vi "LC_Relay_Protection_R2.vi"(0 "Protection settings":T4, 1 "Reset Relay":bool, 3 "RMS minimum\nvalues":cluster{"VRMS values":dbl, "IRMS values":dbl}, 5 "RMS values":dbl[](array[numeric]), 9 "Total power values":dbl[](array[numeric]), 11 "input cluster":T3, 12 "Blocking in":bool, 14 "Transfer Trip":bool) -> (4 "trip signal":bool, 6 "Reclose":bool, 8 "Relay state":cluster{"Lockout":bool, "State":i16}, 10 "Blocking out":bool[](array[boolean]), 15 "output cluster":T3)   [LabVIEW 2016]
doc: "Modified LC_Relay_Protection for Relay2"
uses:
  <vilib>/addons/Electrical Power/Protection/Definite Time Delay/subVIs/fpga_Timer Feedback Var.ctl
  <vilib>/addons/Electrical Power/Protection/Definite Time Delay/subVIs/fpga_State.ctl
  <vilib>/addons/Electrical Power/Protection/Inverse Time Delay/subVIs/ep_Operate Time.ctl
  <vilib>/addons/Electrical Power/Protection/NI_EP_Protection.lvlib
  <vilib>/addons/Electrical Power/Protection/NI_EP_Protection_FPGA.lvlib
panel:
  out "VR error":i32
  out "I error":i32
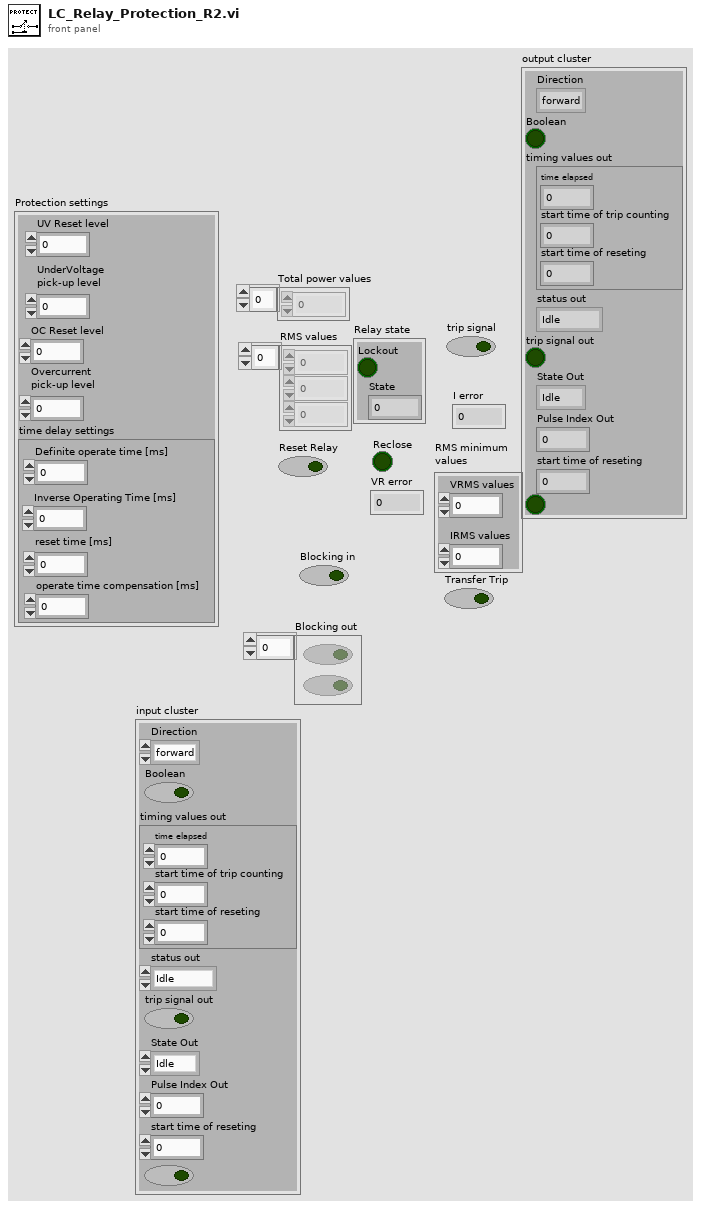
[diagram p1: front panel]
types:
  T1 = typedef "NI_EP_Protection_FPGA.lvlib/fpga_Timer Feedback Var.ctl" = cluster{"time elapsed":u32, "start time of trip counting":u32, "start time of reseting":u32}
  T2 = typedef "NI_EP_Protection_FPGA.lvlib/fpga_State.ctl" = enum16{"Idle", "Trip Counting", "Tripped", "Reset Counting"}
  T3 = cluster{"Direction":enum16{"forward", "backward", "N/D"}, "Boolean":bool, "timing values out":T1, "status out":T2, "trip signal out":bool, "State Out":enum16{"Idle", "Wait for Trip", "PulseClosing", "Locked"}, "Pulse Index Out":i32, "start time of reseting":u32, bool}
  T4 = cluster{"UV Reset level":dbl, "UnderVoltage \npick-up level":dbl, "OC Reset level":dbl, "Overcurrent\npick-up level":dbl, "time delay settings":cluster{"Definite operate time [ms]":u32, "Inverse Operating Time [ms]":u32, "reset time [ms]":u32, "operate time compensation [ms]":u32}}
  T5 = enum16{"Idle", "Wait for Trip", "PulseClosing", "Locked"}
  T6 = cluster{"Definite operate time [ms]":u32, "Inverse Operating Time [ms]":u32, "reset time [ms]":u32, "operate time compensation [ms]":u32}
  T7 = typedef "NI_EP_Protection.lvlib/ep_Operate Time.ctl" = cluster{"A [s]":dbl, "B [s]":dbl, "alpha":dbl, "K2 [s]":dbl, "K1 [s]":dbl, "K3 [s]":dbl}
  T8 = cluster{u32, "reset time [ms]":u32, "reset time [ms]":u32}
  T9 = cluster{"Definite operate time [ms]":u32, "reset time [ms]":u32, "reset time [ms]":u32}
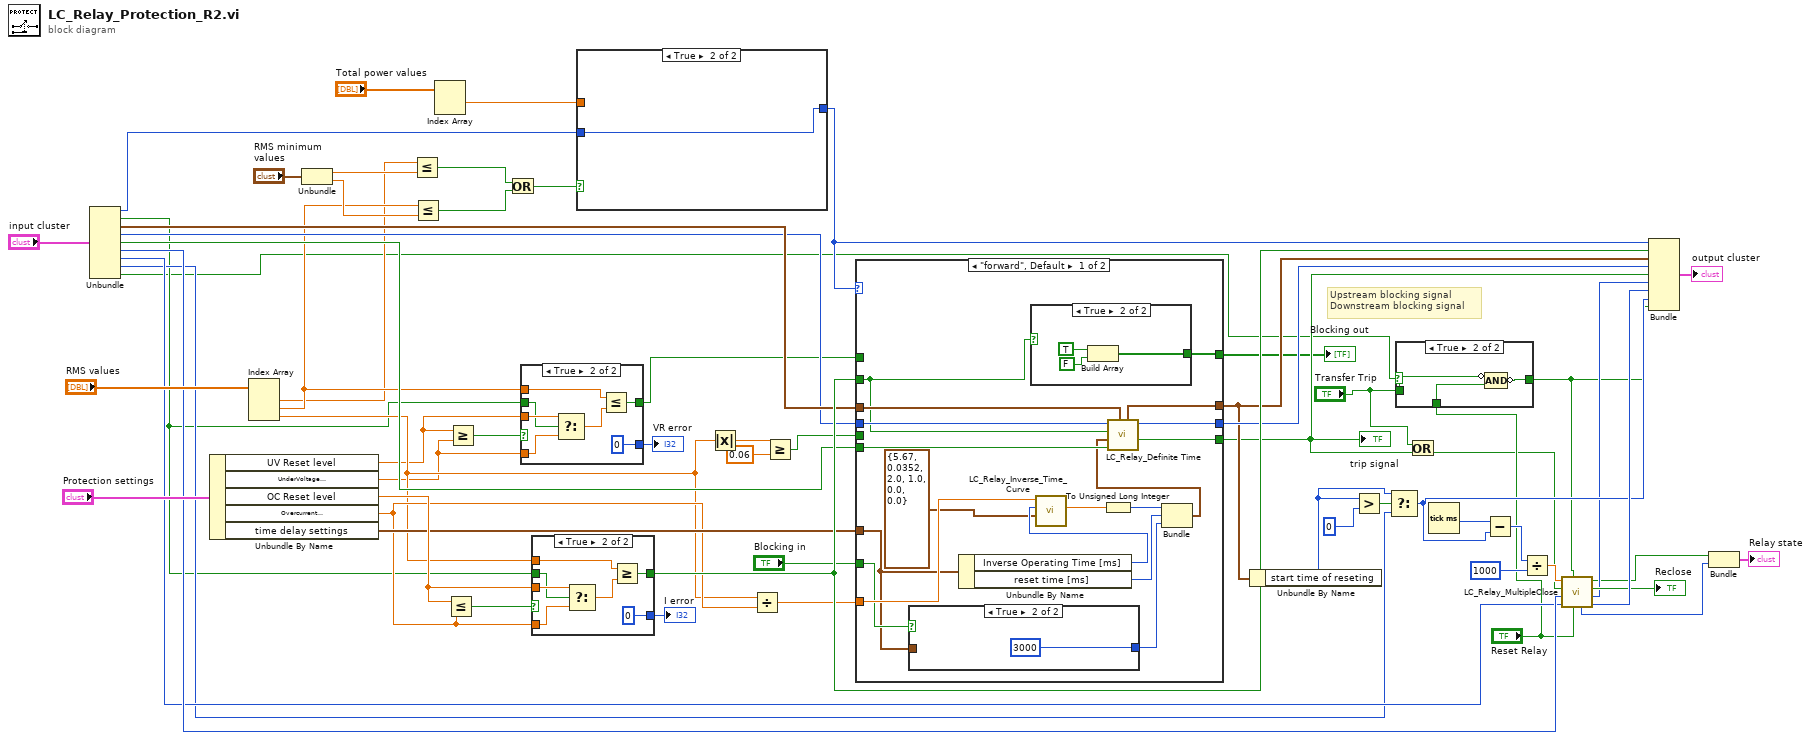
[diagram p0: block diagram]
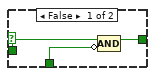
[diagram p2: hidden frame]
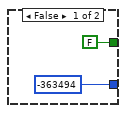
[diagram p3: hidden frame]
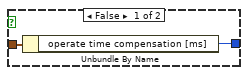
[diagram p4: hidden frame]
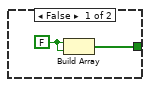
[diagram p5: hidden frame]
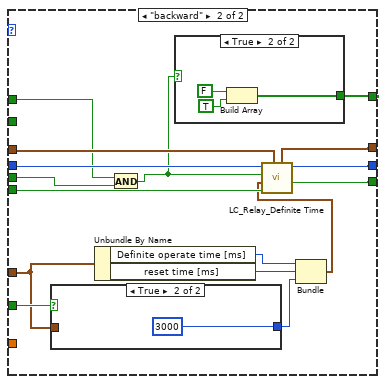
[diagram p6: hidden frame]
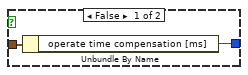
[diagram p7: hidden frame]
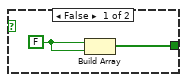
[diagram p8: hidden frame]
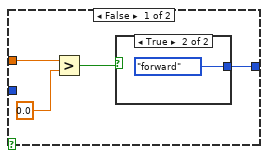
[diagram p9: hidden frame]
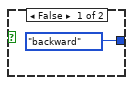
[diagram p10: hidden frame]
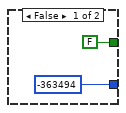
[diagram p11: hidden frame]
diagram:
  # "Upstream blocking signal\nDownstream blocking signal"
  n1 = Unbundle("input cluster") -> ("Direction"=w38:enum16{"forward", "backward", "N/D"}, "Boolean"=w11:bool, "timing values out"=w27:T1, "status out"=w26:T2, "trip signal out"=w25:bool, "State Out"=w24:T5, "Pulse Index Out"=w23:i32, "start time of reseting"=w22:u32, w8:bool)
  n2 = Unbundle By Name("Protection settings") -> ("UV Reset level"=w14:dbl, "UnderVoltage \npick-up level"=w13:dbl, "OC Reset level"=w55:dbl, "Overcurrent\npick-up level"=w40:dbl, "time delay settings"=w53:T6)
  n3 = Index Array(array="RMS values") -> (element #1=w15:dbl, element #2=w21:dbl, element #3=w19:dbl)  [unwired: 3 in]
  n4 = Unbundle("RMS minimum\nvalues") -> ("VRMS values"=w60:dbl, "IRMS values"=w57:dbl)
  n5 = Less Or Equal?(x=w15, y=w60) -> (x <= y?=w59:bool)
  n6 = Less Or Equal?(x=w21, y=w57) -> (x <= y?=w58:bool)
  n7 = Index Array(array="Total power values") -> (element #1=w45:dbl)  [unwired: 2 in, 1 out]
  n8 = Less Or Equal?(x=w55, y=w40) -> (x <= y?=w63:bool)
  n9 = Greater Or Equal?(x=w14, y=w13) -> (x >= y?=w12:bool)
  n10 = Or(x=w59, y=w58) -> (x .or. y?=w50:bool)
  n11 = case shown="True" w12 {
    tunnel: [-363494 ("error") 0 ("error")] -> w28
    tunnel: w14 -> [_ w70]
    tunnel: w13 -> [_ w69]
    tunnel: [FALSE ("Boolean") w68] -> w20
    tunnel: w11 -> [_ w67]
    tunnel: w21 -> [_ w66]
    frame False {
    }
    frame True {
      n12 = Select(t=w70, s=w67, f=w69) -> (s? t:f=w72:dbl)
      n13 = Less Or Equal?(x=w66, y=w72) -> (x <= y?=w68:bool)
    }
  }
  "VR error" <- w28
  n14 = case shown="True" w63 {
    tunnel: [-363494 ("error") 0 ("error")] -> w62
    tunnel: w55 -> [_ w79]
    tunnel: w40 -> [_ w78]
    tunnel: [FALSE ("Boolean") w77] -> w54
    tunnel: w11 -> [_ w76]
    tunnel: w19 -> [_ w75]
    frame False {
    }
    frame True {
      n15 = Select(t=w79, s=w76, f=w78) -> (s? t:f=w81:dbl)
      n16 = Greater Or Equal?(x=w75, y=w81) -> (x >= y?=w77:bool)
    }
  }
  "I error" <- w62
  n17 = case shown="True" w50 {
    tunnel: w45 -> [w83 _]
    tunnel: w38 -> [_ w88]
    tunnel: [w82 w88] -> w37
    frame False {
      n18 = Greater?(x=w83, y=0.0) -> (0:w84:bool)
      n19 = case shown="True" w84 {
        tunnel: [enum16{"forward", "backward"}."backward" enum16{"forward", "backward"}."forward"] -> w82
        frame False {
        }
        frame True {
        }
      }
    }
    frame True {
    }
  }
  n20 = Absolute Value(x=w19) -> (abs(x)=w16:dbl)
  n21 = Divide(x=w19, y=w40) -> (x/y=w51:dbl)
  n22 = Greater Or Equal?(x=w16, y=0.06) -> (x >= y?=w17:bool)
  n23 = case shown="\"forward\", Default" w37 {
    tunnel: w54 -> [w89 _]
    tunnel: w53 -> [w92 w120]
    tunnel: [w106 w125] -> w52
    tunnel: w51 -> [w105 _]
    tunnel: [w104 w126] -> w49
    tunnel: [w90 w124] -> w41
    tunnel: w27 -> [w103 w129]
    tunnel: w26 -> [w102 w128]
    tunnel: w25 -> [w101 w127]
    tunnel: [w94 w123] -> w30
    tunnel: "Blocking in" -> [w93 w122]
    tunnel: w17 -> [_ w115]
    tunnel: w20 -> [_ w117]
    frame "forward", Default {
      n24 = case shown="True" w93 {
        tunnel: [w107 u32 3000 ("reset time [ms]")] -> w91
        tunnel: w92 -> [w108 _]
        frame False {
          n25 = Unbundle By Name(w108) -> ("operate time compensation [ms]"=w107:u32)
        }
        frame True {
        }
      }
      n26 = Unbundle By Name(w92) -> ("Inverse Operating Time [ms]"=w100:u32, "reset time [ms]"=w97:u32)
      n27 = case shown="True" w89 {
        tunnel: [w110 w112] -> w94
        frame False {
          w111 = FALSE
          n28 = Build Array(w111, w111) -> (w110:bool[])
        }
        frame True {
          n29 = Build Array(TRUE, FALSE) -> (w112:bool[])
        }
      }
      n30 = call "LC_Relay_Inverse_Time_Curve.vi"("input cluster"=T7 {"A [s]"=5.67, "B [s]"=0.0352, "alpha"=2.0, "K2 [s]"=1.0, "K1 [s]"=0.0, "K3 [s]"=0.0}, "time dial"=w100, "multiples of pickup"=w105) -> ("oparate time"=w98:dbl)  [unwired: 5 in, 1 out]
      n31 = To Unsigned Long Integer(number=w98) -> (unsigned 32bit integer=w95:u32)
      n32 = Bundle(w95, "reset time [ms]"=w97, "reset time [ms]"=w91) -> (w96:T8)  [unwired: 1 in]
      n33 = call "LC_Relay_Definite Time.vi"("timing values in"=w103, "trip signal in"=w101, "time delay settings"=w96, "pick-up signal? (F)"=w89, "status in"=w102) -> ("trip signal out"=w90:bool, "status out"=w106:T2, "timing values out"=w104:T1)  [unwired: 3 in, 1 out]
    }
    frame "backward" {
      n34 = case shown="True" w122 {
        tunnel: [w131 u32 3000 ("reset time [ms]")] -> w121
        tunnel: w120 -> [w132 _]
        frame False {
          n35 = Unbundle By Name(w132) -> ("operate time compensation [ms]"=w131:u32)
        }
        frame True {
        }
      }
      n36 = Unbundle By Name(w120) -> ("Definite operate time [ms]"=w119:u32, "reset time [ms]"=w130:u32)
      n37 = And(x=w117, y=w115) -> (x .and. y?=w116:bool)
      n38 = case shown="True" w116 {
        tunnel: [w134 w136] -> w123
        frame False {
          w135 = FALSE
          n39 = Build Array(w135, w135) -> (w134:bool[])
        }
        frame True {
          n40 = Build Array(FALSE, TRUE) -> (w136:bool[])
        }
      }
      n41 = Bundle("Definite operate time [ms]"=w119, "reset time [ms]"=w130, "reset time [ms]"=w121) -> (w118:T9)  [unwired: 1 in]
      n42 = call "LC_Relay_Definite Time.vi"("timing values in"=w129, "trip signal in"=w127, "time delay settings"=w118, "pick-up signal? (F)"=w116, "status in"=w128) -> ("trip signal out"=w124:bool, "status out"=w125:T2, "timing values out"=w126:T1)  [unwired: 3 in, 1 out]
    }
  }
  "trip signal" <- w41
  "Blocking out" <- w30
  n43 = Unbundle By Name(w49) -> ("start time of reseting"=w34:u32)
  n44 = Greater?(x=w34, y=u32 0 ("x")) -> (0:w35:bool)
  n45 = Select(t=w34, s=w35, f=w22) -> (s? t:f=w33:u32)
  n46 = case shown="True" w8 {
    tunnel: "Reset Relay" -> [w140 w143]
    tunnel: [w141 w144] -> w7
    tunnel: "Transfer Trip" -> [w139 w142]
    frame False {
      n47 = Compound Arithmetic op=AND(w139, invert w140) -> (w141:bool)
    }
    frame True {
      n48 = Compound Arithmetic op=AND(invert w142, w143) -> (invert w144:bool)
    }
  }
  n49 = Or(x="Transfer Trip", y=w41) -> (x .or. y?=w2:bool)
  n50 = Tick Count (ms)() -> (millisecond timer value=w48:u32)
  n51 = Subtract(x=w48, y=w33) -> (x-y=w43:u32)
  n52 = Divide(x=w43, y=u32 1000) -> (x/y=w32:dbl)
  n53 = call "LC_Relay_MultipleClose.vi"("Reset Relay"="Reset Relay", "Transfer Trip"=w7, "Pulse Index In"=w23, "State In"=w24, "Trip signal"=w2, "Time lapsed"=w32) -> ("Pulse Index Out"=w42:i32, "State Out"=w31:T5, "Reclose"=→"Reclose":bool, "Lockout"=w5:bool, "State"=w4:i16)  [unwired: 1 in]
  n54 = Bundle("Direction"=w37, "Boolean"=w54, "timing values out"=w49, "status out"=w52, "trip signal out"=w41, "State Out"=w31, "Pulse Index Out"=w42, "start time of reseting"=w33, w7) -> (→"output cluster":T3)  [unwired: 1 in]
  n55 = Bundle("Lockout"=w5, "State"=w4) -> (→"Relay state":cluster{"Lockout":bool, "State":i16})  [unwired: 1 in]
